vi "Parse Elements Treewise.vi"(7 "Item Data":refnum<class "Item.lvclass">[](array[class]), 8 "error in":errorcluster, 9 "Parents":string[](array[string]), 10 "XML Info":T2, 11 "Node in":refnum<k20>) -> (0 "error out":errorcluster, 3 "Node out":refnum<k20>, 5 "Item Data out":refnum<class "Item.lvclass">[](array[class]))   [LabVIEW 2020, in "VI Properties Editor.lvlib"]
doc: "Parses the elements of the items contained within <B>XML Info</B>."
uses:
  VI Properties Editor.lvlib
  <vilib>/xml/NI_XML.lvlib
  <vilib>/xml/Close Reference(Node).vi
  Classes/Support/Item Type.ctl
  Classes/Item/Item.lvclass
  CTLs/XPath Get Attribute.ctl
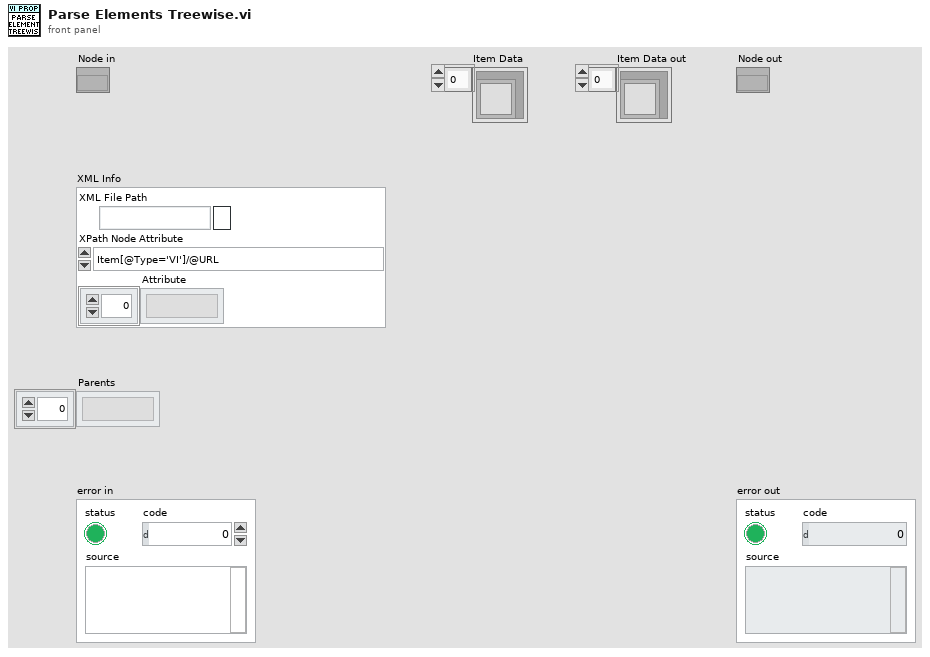
[diagram p1: front panel]
types:
  T1 = typedef "VI Properties Editor.lvlib/XPath Get Attribute.ctl" = enum16{"Item[@Type='VI']/@URL", "Item[@Type='LVClass']/@URL", "Item[@Type='Library']/@URL", "Item[@Type='Folder' and not (@URL)]/@Name", "@Name"}
  T2 = cluster{"XML File Path":path, "XPath Node Attribute":T1, "Attribute":string[]}
  T3 = typedef "VI Properties Editor.lvlib/Item Type.ctl" = enum16{"Generic", "VI"}
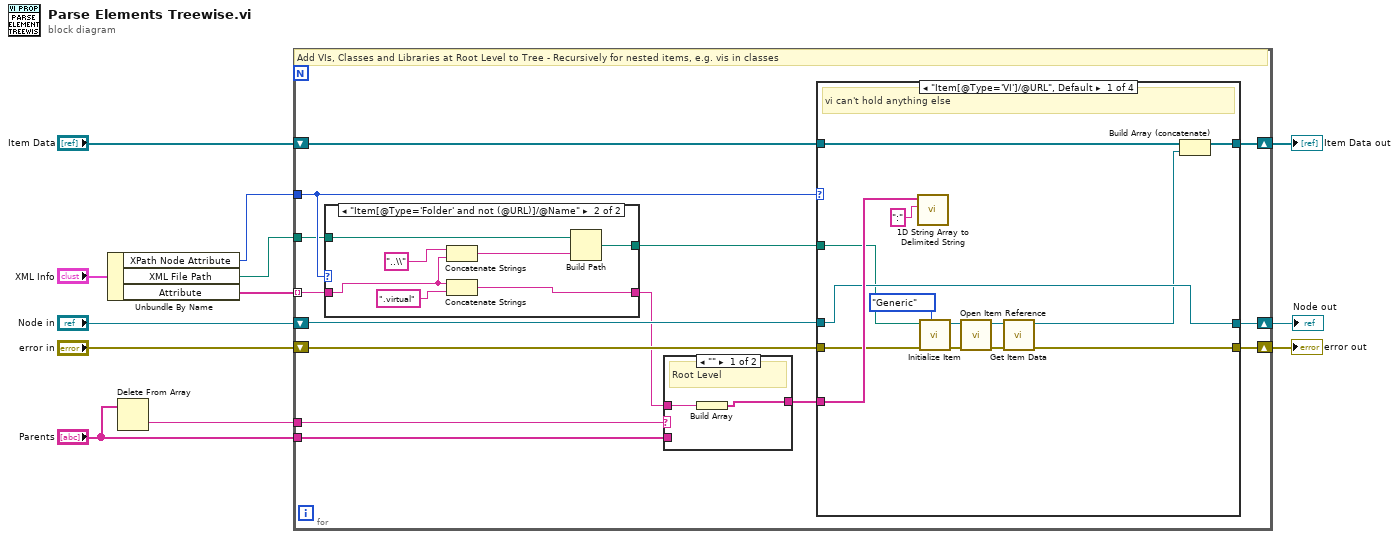
[diagram p0: block diagram]
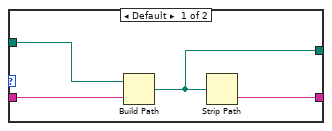
[diagram p2: hidden frame]
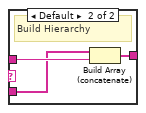
[diagram p3: hidden frame]
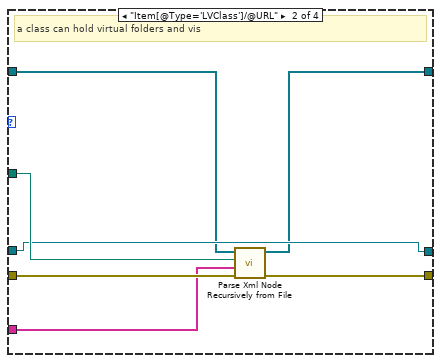
[diagram p4: hidden frame]
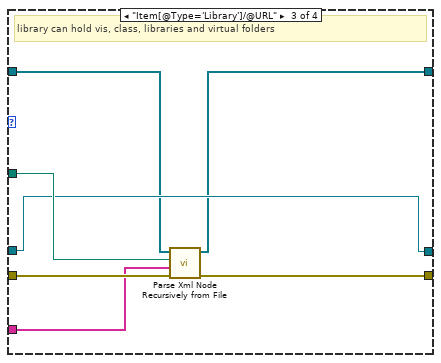
[diagram p5: hidden frame]
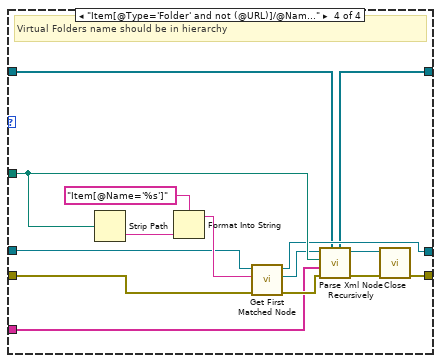
[diagram p6: hidden frame]
diagram:
  n1 = Unbundle By Name("XML Info") -> ("XPath Node Attribute"=w2:T1, "XML File Path"=w3:path, "Attribute"=w1:string[])
  n2 = Delete From Array(array="Parents") -> (deleted portion=w6:string)  [unwired: 2 in, 1 out]
  n3 = for {
    shift-right: [w26] -> w8
    shift-left: "error in" -> [w20]
    tunnel: w2 -> [w18]
    tunnel: w3 -> [w15]
    tunnel: w1 -> [w16] mode=indexing
    tunnel: "Parents" -> [w21]
    shift-right: [w24] -> w11
    shift-left: "Item Data" -> [w23]
    tunnel: w6 -> [w22]
    shift-right: [w13] -> w5
    shift-left: "Node in" -> [w19]
    # "Add VIs, Classes and Libraries at Root Level to Tree - Recursively for nested items, e.g. vis in classes"
    n4 = case shown="\"Item[@Type='Folder' and not (@URL)]/@Name\"" w18 {
      tunnel: w16 -> [w29 w35]
      tunnel: [w28 w36] -> w17
      tunnel: w15 -> [w30 w33]
      tunnel: [w27 w31] -> w14
      frame Default {
        n5 = Build Path(base path=w30, name or relative path=w29) -> (appended path=w27:path)
        n6 = Strip Path(path=w27) -> (name=w28:string)  [unwired: 1 out]
      }
      frame "Item[@Type='Folder' and not (@URL)]/@Name" {
        # "Virtual F."
        n7 = Concatenate Strings("..\\" ("string"), w35) -> (w32:string)
        n8 = Concatenate Strings(w35, ".virtual" ("string")) -> (w36:string)
        n9 = Build Path(base path=w33, name or relative path=w32) -> (appended path=w31:path)
      }
    }
    n10 = case shown="\"\"" w22 {
      tunnel: w17 -> [w39 w42]
      tunnel: [w38 w41] -> w25
      tunnel: w21 -> [_ w40]
      frame "" {
        # "Root Level"
        n11 = Build Array(w39) -> (w38:string[])
      }
      frame Default {
        # "Build Hierarchy"
        n12 = Build Array (concatenate)(w40, w42) -> (w41:string[])
      }
    }
    n13 = case shown="\"Item[@Type='VI']/@URL\", Default" w18 {
      tunnel: [w56 w63 w69 w84] -> w26
      tunnel: w20 -> [w50 w62 w70 w80]
      tunnel: w14 -> [w47 w61 w68 w78]
      tunnel: w25 -> [w54 w60 w67 w73]
      tunnel: [w52 w57 w64 w71] -> w24
      tunnel: w23 -> [w53 w58 w65 w72]
      tunnel: w19 -> [w51 w59 w66 w81]
      tunnel: [w51 w59 w66 w74] -> w13
      frame "Item[@Type='VI']/@URL", Default {
        # "vi can't hold anything else"
        n14 = call <vilib>:"1D String Array to Delimited String.vi"("delimiter"=":", "string array"=w54) -> ()  [unwired: 9 in, 1 out]
        n15 = call "Initialize Item.vi"("Item Type"=Item_Type."Generic", "error in (no error)"=w50, "Path"=w47) -> ("error out"=w49:errorcluster, "Item"=w46:refnum<class "Item.lvclass">)  [unwired: 7 in]
        n16 = call-dynamic "Open Item Reference.vi"("error in (no error)"=w49, "Item in"=w46) -> ("error out"=w45:errorcluster, "Item out"=w44:refnum<class "Item.lvclass">)  [unwired: 8 in]
        n17 = call-dynamic "Get Item Data.vi"("error in (no error)"=w45, "Item in"=w44) -> ("error out"=w56:errorcluster, "Item out"=w43:refnum<class "Item.lvclass">)  [unwired: 8 in]
        n18 = Build Array (concatenate)(w53, w43) -> (w52:refnum<class "Item.lvclass">[])
      }
      frame "Item[@Type='LVClass']/@URL" {
        # "a class can hold virtual folders and vis"
        n19 = call "Parse Xml Node Recursively from File.vi"("error in"=w62, "Parents"=w60, "Path to XML document"=w61, "Item Data"=w58) -> ("error out"=w63:errorcluster, "Item Data out"=w57:refnum<class "Item.lvclass">[])  [unwired: 6 in]
      }
      frame "Item[@Type='Library']/@URL" {
        # "library can hold vis, class, libraries and virtual folders"
        n20 = call "Parse Xml Node Recursively from File.vi"("error in"=w70, "Parents"=w67, "Path to XML document"=w68, "Item Data"=w65) -> ("error out"=w69:errorcluster, "Item Data out"=w64:refnum<class "Item.lvclass">[])  [unwired: 6 in]
      }
      frame "Item[@Type='Folder' and not (@URL)]/@Name" {
        # "Virtual Folders name should be in hierarchy"
        n21 = Strip Path(path=w78) -> (name=w77:string)  [unwired: 1 out]
        n22 = Format Into String(format string="Item[@Name='%s']" ("XPath expression"), w77) -> (resulting string=w82:string)  [unwired: 2 in, 1 out]
        n23 = call <vilib>:"Get First Matched Node.vi"("error in (no error)"=w80, "XPath expression"=w82, "node in"=w81) -> ("error out"=w79:errorcluster, "node result"=w76:refnum<k20>, "node out"=w74:refnum<k20>)  [unwired: 6 in]
        n24 = call "Parse Xml Node Recursively.vi"("Item Data"=w72, "error in"=w79, "Parents"=w73, "XML File Path"=w78, "Node in"=w76) -> ("error out"=w85:errorcluster, "Node out"=w75:refnum<k20>, "Item Data out"=w71:refnum<class "Item.lvclass">[])  [unwired: 4 in]
        n25 = call-poly <vilib>:"Close.vi"("error in (no error)"=w85, "node"=w75) -> ("error out"=w84:errorcluster)  [unwired: 7 in]
      }
    }
  }
  "Item Data out" <- w11
  "error out" <- w8
  "Node out" <- w5
